vi "Tachomodus (SubVI).vi"(0 "Lambda":refnum<vi>, 4 "Temp":refnum<vi>, 5 "AFR EGT":refnum<vi>, 6 "AFR":refnum<vi>, 7 "cvt":bool, 8 "Leistung":refnum<vi>, 9 "Stopp":refnum<vi>, 10 "Hinterrad":refnum<vi>, 11 "Welle":refnum<vi>) -> ()   [LabVIEW 2014]
panel:
  in  "Reset":bool
  out "°Cmax":dbl format="%#.0f"
  out "AFRmax":dbl format="%.1f"
  in  "Text Rolle":string="Dyno"
  in  "Text Zündung":string="Ignition"
  out "Welle [1/min]\n[1/min]":cluster{dbl, dbl}(knob) caption="Engine\n[1/min]" scale=0.0..14000.0
  out "Hinterrad (Tacho)\n[km/h]":dbl(knob) caption="Rear Tire\n[km/h]" scale=0.0..200.0
  out "[°C]":dbl
  out "AFR":dbl format="%.1f"
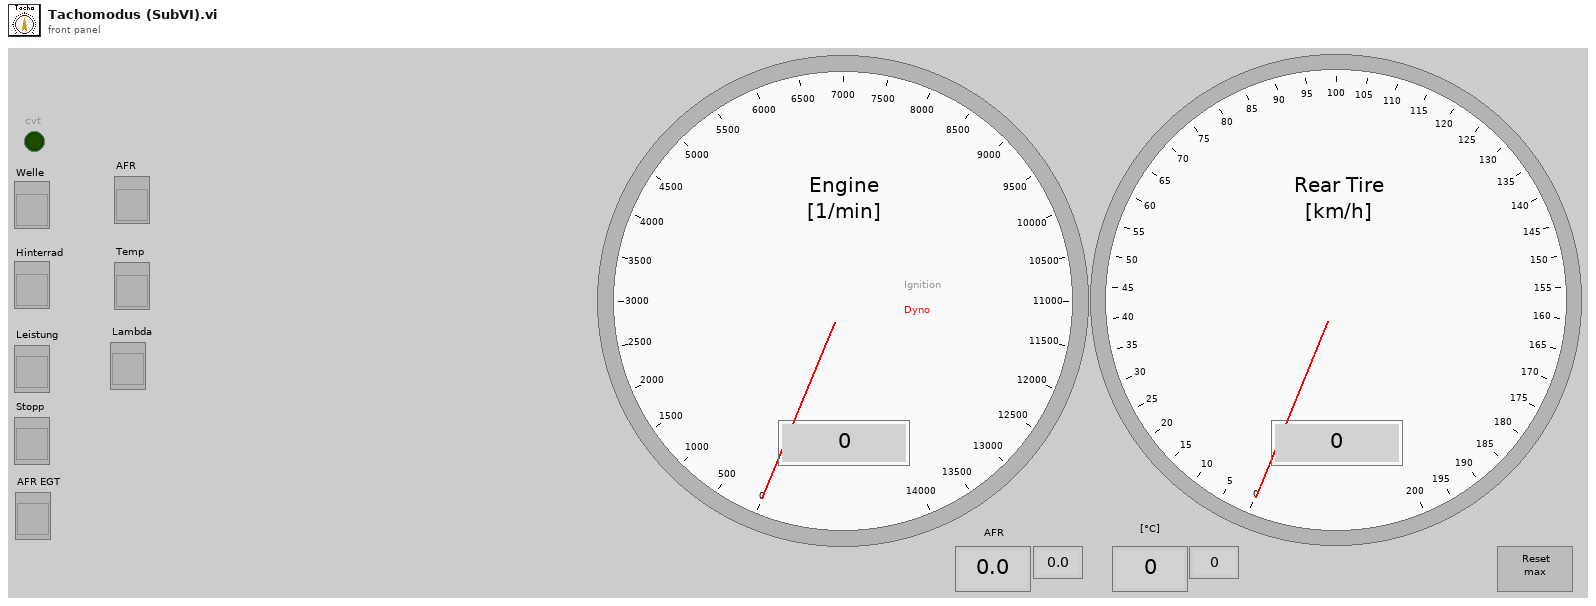
[diagram p1: front panel]
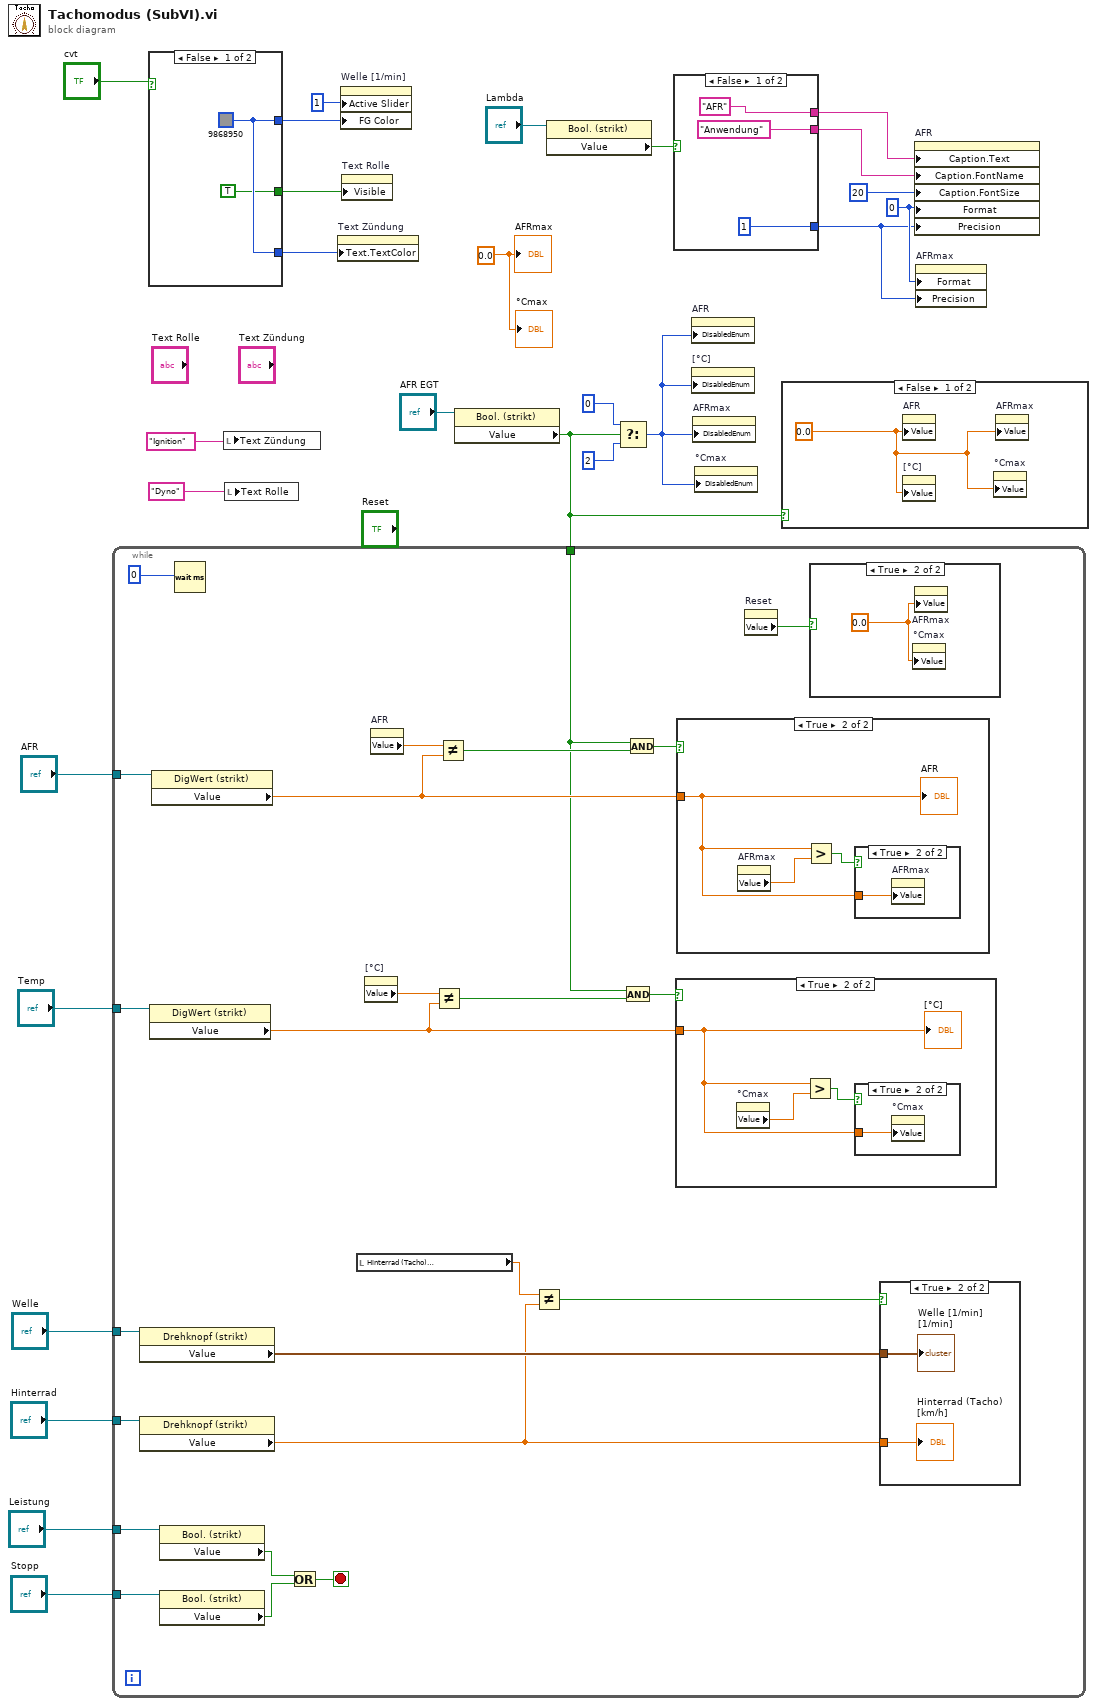
[diagram p0: block diagram]
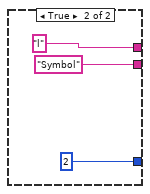
[diagram p3: hidden frame]
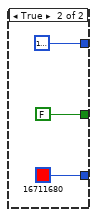
[diagram p4: hidden frame]
diagram:
  w4 = 0.0
  w2 = 0
  n1 = case shown="False" "cvt" {
    tunnel: [w28 u32 16711680] -> w17
    tunnel: [w28 u32 16777216] -> w19
    tunnel: [TRUE FALSE] -> w20
    frame False {
      w28 = u32 9868950
    }
    frame True {
    }
  }
  n2 = local write "Text Zündung"("Ignition") -> ()
  n3 = local write "Text Rolle"("Dyno") -> ()
  n4 = property on="Text Zündung" class="Str"("Text.TextColor"=w17) -> ()  [unwired: 2 in, 2 out]
  n5 = property on="Welle [1/min]" class="Drehknopf (strikt)"("Active Slider"=1, "FG Color"=w19) -> ()  [unwired: 2 in, 2 out]
  n6 = property on="Text Rolle" class="Str"("Visible"=w20) -> ()  [unwired: 2 in, 2 out]
  n7 = property class="Bool. (strikt)"(reference="AFR EGT") -> ("Value"=w7:bool)  [unwired: 1 in, 2 out]
  n8 = while {
    tunnel: "Welle" -> [w55]
    tunnel: "Hinterrad" -> [w54]
    tunnel: "Leistung" -> [w53]
    tunnel: "Stopp" -> [w51]
    tunnel: w7 -> [w32]
    tunnel: "AFR" -> [w43]
    tunnel: "Temp" -> [w42]
    stop <- w48 stop-if-true
    n9 = property class="Drehknopf (strikt)"(reference=w55) -> ("Value"=w49:cluster{dbl, dbl})  [unwired: 1 in, 2 out]
    n10 = property class="Drehknopf (strikt)"(reference=w54) -> ("Value"=w44:dbl)  [unwired: 1 in, 2 out]
    n11 = property class="DigWert (strikt)"(reference=w42) -> ("Value"=w33:dbl)  [unwired: 1 in, 2 out]
    n12 = property class="DigWert (strikt)"(reference=w43) -> ("Value"=w39:dbl)  [unwired: 1 in, 2 out]
    n13 = property class="Bool. (strikt)"(reference=w53) -> ("Value"=w52:bool)  [unwired: 1 in, 2 out]
    n14 = property class="Bool. (strikt)"(reference=w51) -> ("Value"=w50:bool)  [unwired: 1 in, 2 out]
    n15 = Wait (ms)(milliseconds to wait=0) -> ()  [unwired: 1 out]
    n16 = Or(x=w52, y=w50) -> (x .or. y?=w48:bool)
    n17 = local read "Hinterrad (Tacho)\n[km/h]"() -> (w45:dbl)
    n18 = property on="[°C]" class="DigWert (strikt)"() -> ("Value"=w35:dbl)  [unwired: 2 in, 2 out]
    n19 = property on="AFR" class="DigWert (strikt)"() -> ("Value"=w40:dbl)  [unwired: 2 in, 2 out]
    n20 = Not Equal?(x=w35, y=w33) -> (x != y?=w36:bool)
    n21 = Not Equal?(x=w40, y=w39) -> (x != y?=w37:bool)
    n22 = Not Equal?(x=w45, y=w44) -> (x != y?=w46:bool)
    n23 = And(x=w32, y=w36) -> (x .and. y?=w34:bool)
    n24 = And(x=w32, y=w37) -> (x .and. y?=w38:bool)
    n25 = case shown="True" w34 {
      tunnel: w33 -> [_ w58]
      frame False {
      }
      frame True {
        n26 = property on="°Cmax" class="DigWert (strikt)"() -> ("Value"=w56:dbl)  [unwired: 2 in, 2 out]
        n27 = Greater?(x=w58, y=w56) -> (0:w57:bool)
        n28 = case shown="True" w57 {
          tunnel: w58 -> [_ w59]
          frame False {
          }
          frame True {
            n29 = property on="°Cmax" class="DigWert (strikt)"("Value"=w59) -> ()  [unwired: 2 in, 2 out]
          }
        }
        "[°C]" <- w58
      }
    }
    n30 = case shown="True" w38 {
      tunnel: w39 -> [_ w62]
      frame False {
      }
      frame True {
        n31 = property on="AFRmax" class="DigWert (strikt)"() -> ("Value"=w60:dbl)  [unwired: 2 in, 2 out]
        n32 = Greater?(x=w62, y=w60) -> (0:w61:bool)
        n33 = case shown="True" w61 {
          tunnel: w62 -> [_ w63]
          frame False {
          }
          frame True {
            n34 = property on="AFRmax" class="DigWert (strikt)"("Value"=w63) -> ()  [unwired: 2 in, 2 out]
          }
        }
        "AFR" <- w62
      }
    }
    n35 = property on="Reset" class="Bool. (strikt)"() -> ("Value"=w41:bool)  [unwired: 2 in, 2 out]
    n36 = case shown="True" w41 {
      frame False {
      }
      frame True {
        w64 = 0.0
        n37 = property on="°Cmax" class="DigWert (strikt)"("Value"=w64) -> ()  [unwired: 2 in, 2 out]
        n38 = property on="AFRmax" class="DigWert (strikt)"("Value"=w64) -> ()  [unwired: 2 in, 2 out]
      }
    }
    n39 = case shown="True" w46 {
      tunnel: w49 -> [_ w66]
      tunnel: w44 -> [_ w65]
      frame False {
      }
      frame True {
        "Welle [1/min]\n[1/min]" <- w66
        "Hinterrad (Tacho)\n[km/h]" <- w65
      }
    }
  }
  n40 = property class="Bool. (strikt)"(reference="Lambda") -> ("Value"=w12:bool)  [unwired: 1 in, 2 out]
  n41 = Select(t=0, s=w7, f=2) -> (s? t:f=w3:i32)
  n42 = case shown="False" w12 {
    tunnel: ["AFR" "l"] -> w13
    tunnel: ["Anwendung" "Symbol"] -> w14
    tunnel: [1 2] -> w1
    frame False {
    }
    frame True {
    }
  }
  n43 = property on="AFR" class="DigWert (strikt)"("DisabledEnum"=w3) -> ()  [unwired: 2 in, 2 out]
  n44 = property on="[°C]" class="DigWert (strikt)"("DisabledEnum"=w3) -> ()  [unwired: 2 in, 2 out]
  n45 = property on="AFRmax" class="DigWert (strikt)"("DisabledEnum"=w3) -> ()  [unwired: 2 in, 2 out]
  n46 = property on="°Cmax" class="DigWert (strikt)"("DisabledEnum"=w3) -> ()  [unwired: 2 in, 2 out]
  n47 = case shown="False" w7 {
    frame False {
      w73 = 0.0
      n48 = property on="AFR" class="DigWert (strikt)"("Value"=w73) -> ()  [unwired: 2 in, 2 out]
      n49 = property on="[°C]" class="DigWert (strikt)"("Value"=w73) -> ()  [unwired: 2 in, 2 out]
      n50 = property on="°Cmax" class="DigWert (strikt)"("Value"=w73) -> ()  [unwired: 2 in, 2 out]
      n51 = property on="AFRmax" class="DigWert (strikt)"("Value"=w73) -> ()  [unwired: 2 in, 2 out]
    }
    frame True {
    }
  }
  n52 = property on="AFR" class="DigWert (strikt)"("Caption.Text"=w13, "Caption.FontName"=w14, "Caption.FontSize"=20, "Format"=w2, "Precision"=w1) -> ()  [unwired: 2 in, 2 out]
  n53 = property on="AFRmax" class="DigWert (strikt)"("Format"=w2, "Precision"=w1) -> ()  [unwired: 2 in, 2 out]
  "AFRmax" <- w4
  "°Cmax" <- w4
